vi "Set_Names_ID_Users.vi"(8 "error in (no error)":errorcluster, 11 "DB in":refnum<class "DB.lvclass">) -> (0 "error out":errorcluster, 3 "DB out":refnum<class "DB.lvclass">)   [LabVIEW 2015, in "DB.lvclass"]
uses:
  DB.lvclass
  DB.lvclass/DB.ctl
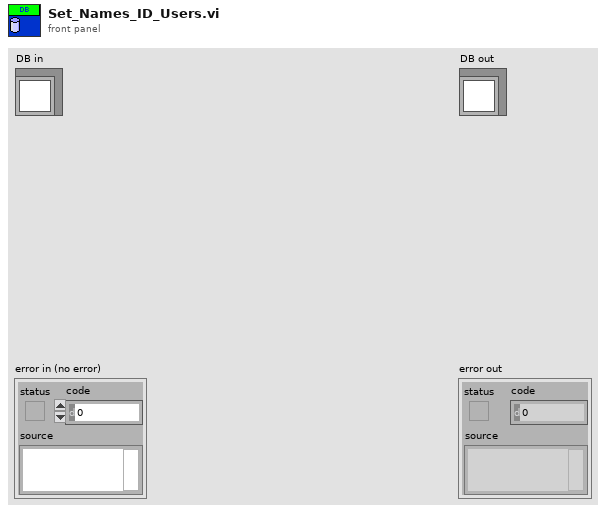
[diagram p1: front panel]
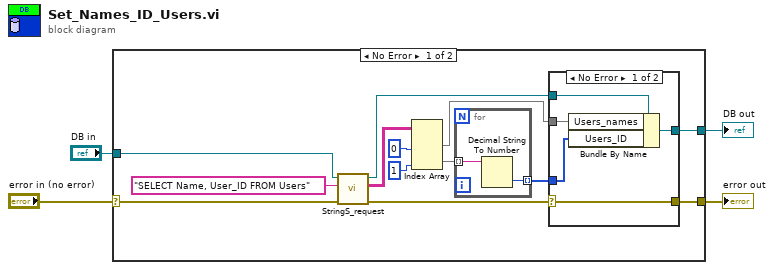
[diagram p0: block diagram]
diagram:
  n1 = case shown="No Error" "error in (no error)" {
    selector: "error in (no error)" -> [w6 w28]
    tunnel: [w8 w28] -> w3
    tunnel: [w9 w27] -> w1
    tunnel: "DB in" -> [w7 w27]
    frame No Error {
      n2 = call-dynamic "StringS_request.vi"("error in (no error)"=w6, "SQL request"="SELECT Name, User_ID FROM Users" ("SQL"), "DB in"=w7) -> ("error out"=w15:errorcluster, "Result Set"=w13:string[][], "DB out"=w17:refnum<class "DB.lvclass">)  [unwired: 5 in, 1 out]
      n3 = Index Array(array=w13, index (col) #1=0 ("disabled index (col)"), index (col) #2=1 ("index (col)")) -> (element #1=w16:string[], element #2=w12:string[])  [unwired: 2 in]
      n4 = for {
        tunnel: w12 -> [w26] mode=indexing
        tunnel: [w25] -> w14 mode=indexing
        n5 = Decimal String To Number(string=w26) -> (number=w25:i32)  [unwired: 2 in, 1 out]
      }
      n6 = case shown="No Error" w15 {
        selector: w15 -> [w18 w23]
        tunnel: w17 -> [w22 w24]
        tunnel: [w21 w24] -> w9
        tunnel: w14 -> [w20 _]
        tunnel: w16 -> [w19 _]
        tunnel: [w18 w23] -> w8
        frame No Error {
          n7 = Bundle By Name(cluster=w22, "Users_names"=w19, "Users_ID"=w20) -> (w21:refnum<class "DB.lvclass">)
        }
        frame Error {
        }
      }
    }
    frame Error {
    }
  }
  "error out" <- w3
  "DB out" <- w1
